vi "Calibration Cal Execute Get Cal Executed.vi"(8 "error in (no error)":errorcluster, 11 "niDTS Calibration Cal Execute RF Test in":refnum<class "niDTS Calibration Cal Execute RF Test.lvclass">) -> (0 "error out":errorcluster, 2 "Cal Executed":bool, 3 "niDTS Calibration Cal Execute RF Test out":refnum<class "niDTS Calibration Cal Execute RF Test.lvclass">)   [LabVIEW 2015, in "niDTS Utilities.lvlib" / "niDTS Calibration Cal Execute RF Test.lvclass"]
uses:
  niDTS Calibration Cal Execute RF Test.lvclass
  niDTS Calibration Cal Execute RF Test.lvclass/niDTS Calibration Cal Execute RF Test.ctl
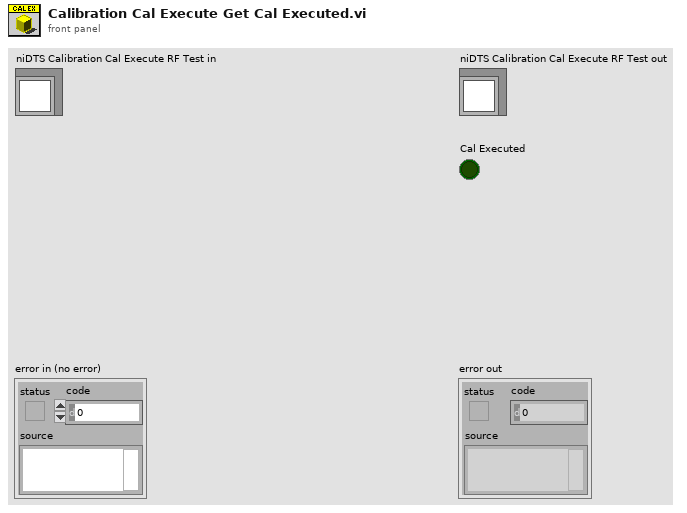
[diagram p1: front panel]
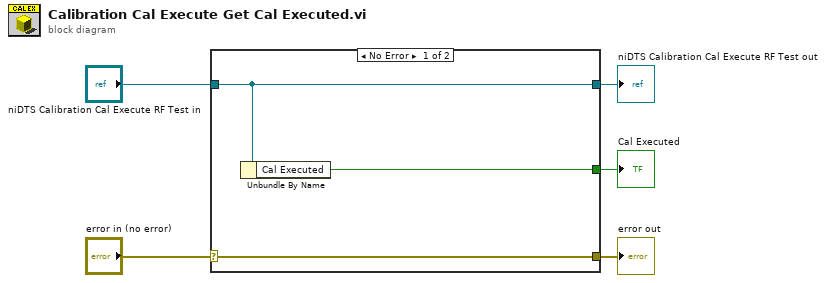
[diagram p0: block diagram]
diagram:
  n1 = case shown="No Error" "error in (no error)" {
    selector: "error in (no error)" -> [w8 w9]
    tunnel: [w8 w9] -> w4
    tunnel: [w7 w10] -> w2
    tunnel: "niDTS Calibration Cal Execute RF Test in" -> [w7 w10]
    tunnel: [w6 _] -> w1
    frame No Error {
      n2 = Unbundle By Name(w7) -> ("Cal Executed"=w6:bool)
    }
    frame Error {
    }
  }
  "error out" <- w4
  "niDTS Calibration Cal Execute RF Test out" <- w2
  "Cal Executed" <- w1
